vi "copy user model VI.vi"(8 "error in":errorcluster, 10 "project directory":path, 11 "VI path":path) -> (0 "error out":errorcluster, 3 "new VI path":path)   [LabVIEW 2014, in "CD model script.lvlib"]
uses:
  CD model script.lvlib
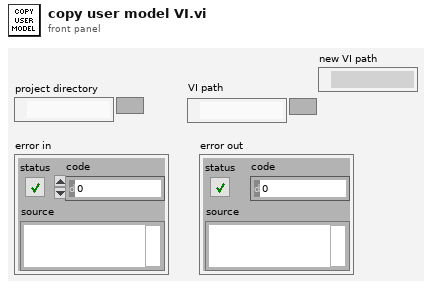
[diagram p1: front panel]
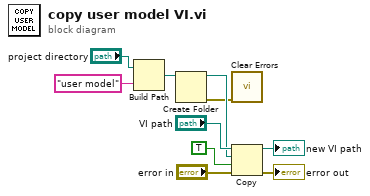
[diagram p0: block diagram]
diagram:
  n1 = Build Path(base path="project directory", name or relative path="user model") -> (appended path=w3:path)
  n2 = Create Folder(path (use dialog)=w3) -> (created path=w2:path, error out=w1:errorcluster)  [unwired: 2 in, 1 out]
  n3 = call <vilib>:"Clear Errors.vi"("error in (no error)"=w1) -> ()  [unwired: 5 in, 2 out]
  n4 = Copy(8:"error in", 9:TRUE ("overwrite (F)"), 10:w2, 11:"VI path") -> (0:→"error out":errorcluster, 3:→"new VI path":path)  [unwired: 1 in, 1 out]
